vi "RisingEdge.vi"(11 "BooleanIn":bool=TRUE) -> (3 "BooleanOut":bool)   [LabVIEW 2012]
doc: "Outputs true only if the previous instance of BooleanIn is false and the current instance of BooleanIn is true, otherwise outputs false (the first call to this VI will always return false)."
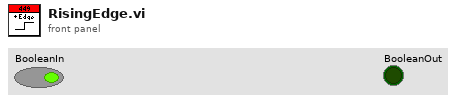
[diagram p1: front panel]
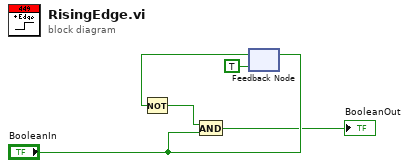
[diagram p0: block diagram]
diagram:
  n1 = feedback-in #1("BooleanIn") -> ()
  n2 = feedback #1(TRUE ("BooleanIn")) -> (w5:bool)
  n3 = Not(x=w5) -> (.not. x?=w4:bool)
  n4 = And(x=w4, y="BooleanIn") -> (x .and. y?=→"BooleanOut":bool)
